vi "Get Posic Motor Indexer.vi"(1 "Controlador":u16(ring)=1 items=["ZERO", "AH", "DEC", "TUBO", "CUP"]) -> (0 "PosMotor":dbl)   [LabVIEW 2018]
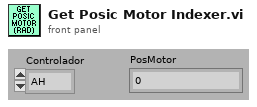
[diagram p1: front panel]
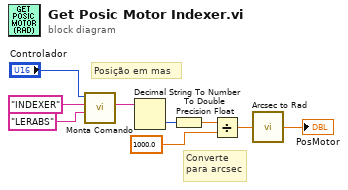
[diagram p0: block diagram]
diagram:
  # "Converte\npara arcsec"
  # "Posição em mas"
  n1 = call "Monta Comando.vi"("Comando"="LERABS", "Dispositivo"="INDEXER" ("Comando"), "Controlador"="Controlador") -> ("Resposta"=w6:string)  [unwired: 3 in, 3 out]
  n2 = Decimal String To Number(string=w6) -> (number=w5:i32)  [unwired: 2 in, 1 out]
  n3 = To Double Precision Float(number=w5) -> (double precision float=w4:dbl)
  n4 = Divide(x=w4, y=1000.0) -> (x/y=w2:dbl)
  n5 = call "Arcsec to Rad.vi"("Arcsec"=w2) -> ("rad"=→"PosMotor":dbl)
